vi "4.vi"() -> ()   [LabVIEW 2017]
panel:
  out "XY图":cluster{cluster{"x2":dbl, "y2":dbl}[]}[](graph)
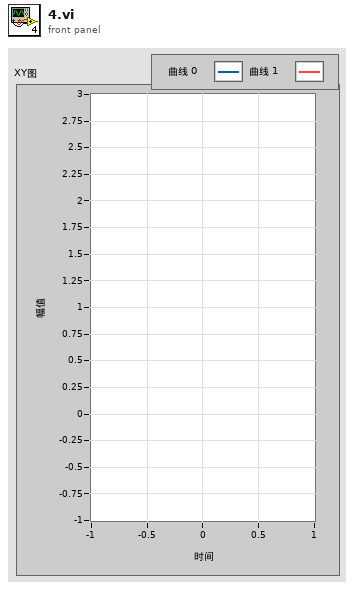
[diagram p1: front panel]
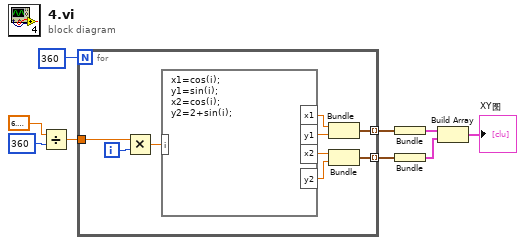
[diagram p0: block diagram]
diagram:
  n1 = Divide(x=6.283185307179586, y=360) -> (x/y=w6:dbl)
  n2 = for {
    N: 360 -> [_]
    tunnel: w6 -> [w15]
    tunnel: [w11] -> w5 mode=indexing
    tunnel: [w10] -> w4 mode=indexing
    i -> [w16]
    n3 = Multiply(x=w15, y=w16) -> (x*y=w14:dbl)
    n4 = formula code="x1=cos(i);\ny1=sin(i);\nx2=cos(i);\ny2=2+sin(i);"("i"=w14) -> ("x1"=w18:dbl, "x2"=w13:dbl, "y1"=w17:dbl, "y2"=w12:dbl)
    n5 = Bundle("x1"=w18, "y1"=w17) -> (w11:cluster{"x1":dbl, "y1":dbl})  [unwired: 1 in]
    n6 = Bundle("x2"=w13, "y2"=w12) -> (w10:cluster{"x2":dbl, "y2":dbl})  [unwired: 1 in]
  }
  n7 = Bundle(w5) -> (w3:cluster{cluster{"x1":dbl, "y1":dbl}[]})  [unwired: 1 in]
  n8 = Bundle(w4) -> (w2:cluster{cluster{"x2":dbl, "y2":dbl}[]})  [unwired: 1 in]
  n9 = Build Array(w3, w2) -> (→"XY图":cluster{cluster{"x2":dbl, "y2":dbl}[]}[])
